vi "Batch Dataset Retrieval.vi"(8 "error in":errorcluster, 11 "Transactions":T1[](array[typedef])) -> (0 "error out":errorcluster, 3 "Data":dbl[][](array[numeric]))   [LabVIEW 2009]
uses:
  Dataset Transaction Id.ctl
  Dataset Source.ctl
  Dataset Type.ctl
  Apps/Yes No Button.ctl
  Data Access Objects/Metadata/DAO Actions.ctl
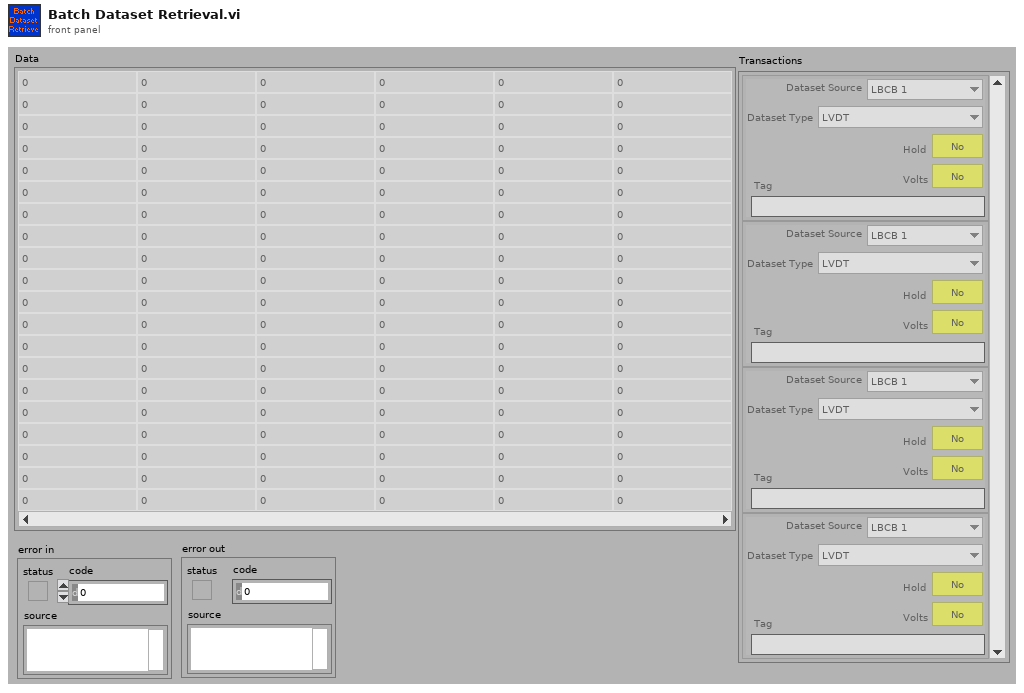
[diagram p1: front panel]
types:
  T1 = typedef "Dataset Transaction Id.ctl" = cluster{"Dataset Source":T2, "Dataset Type":T3, "Hold":T4, "Volts":T4, "Tag":string}
  T2 = typedef "Dataset Source.ctl" = enum16{"LBCB 1", "LBCB 2", "Combined", "External Sensors"}
  T3 = typedef "Dataset Type.ctl" = enum16{"LVDT", "Load Cell", "Actuator Command", "Servo Error", "Displacement Command", "Displacement", "Force"}
  T4 = typedef "Yes No Button.ctl" = bool
  T5 = typedef "DAO Actions.ctl" = enum16{"Init", "Get", "Set"}
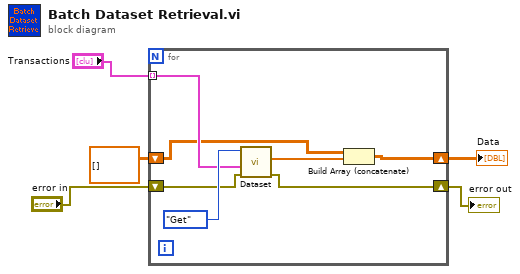
[diagram p0: block diagram]
diagram:
  n1 = for {
    shift-right: [w10] -> w2
    shift-left: "error in" -> [w9]
    tunnel: "Transactions" -> [w8] mode=indexing
    shift-right: [w7] -> w4
    shift-left: dbl[][] [] -> [w6]
    n2 = call "Dataset.vi"("error in (no error)"=w9, "Dataset Trans Id"=w8, "DAO Actions"=DAO_Actions."Get") -> ("error out"=w10:errorcluster, "Data Out"=w12:dbl[])  [unwired: 7 in]
    n3 = Build Array (concatenate)(w6, w12) -> (w7:dbl[][])
  }
  "Data" <- w4
  "error out" <- w2
